vi "Stage Conditional Convert to TDMS.vi"(8 "error in (no error)":errorcluster, 11 "input cluster":T1={"Test_File"=path "", "Status"="Done", "RF_Center_Freq"=0.0, "RF_Gain"=0.0, "BB_Gain"=0.0, "Error 2"="", "file_max"=0, "file_index"=0}) -> (0 "error out":errorcluster, 2 "Converted Binary to TDMS location":path, 3 "output cluster":T1={"Test_File"=path "", "Status"="Done", "RF_Center_Freq"=0.0, "RF_Gain"=0.0, "BB_Gain"=0.0, "Error 2"="", "file_max"=0, "file_index"=0})   [LabVIEW 2017]
uses:
  TypeDef/ESC Internal Data Structure (types).ctl
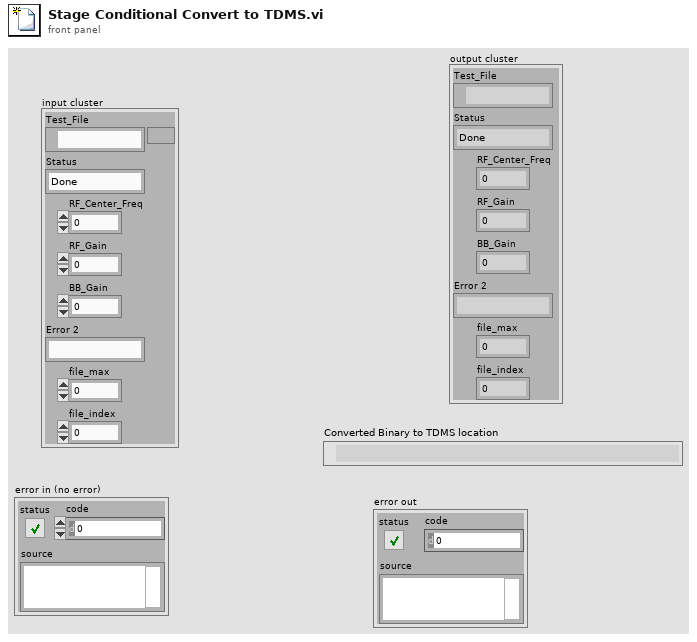
[diagram p1: front panel]
types:
  T1 = typedef "ESC Internal Data Structure (types).ctl" = cluster{"Test_File":path, "Status":string, "RF_Center_Freq":dbl, "RF_Gain":dbl, "BB_Gain":dbl, "Error 2":string, "file_max":u64, "file_index":u64}
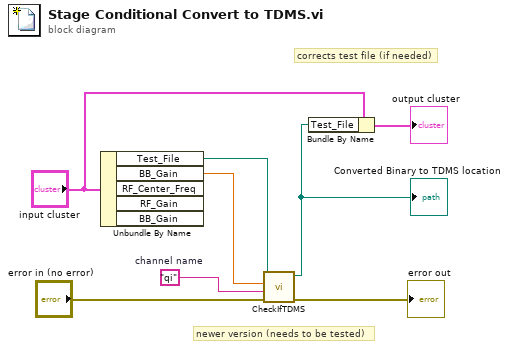
[diagram p0: block diagram]
diagram:
  w6 = "qi"  # channel name
  # "newer version (needs to be tested)"
  # "corrects test file (if needed)"
  n1 = Unbundle By Name("input cluster") -> ("Test_File"=w8:path, "BB_Gain"=w7:dbl)  [unwired: 3 out]
  n2 = call "CheckIfTDMS.vi"("error in (no error)"="error in (no error)", "channel name"=w6, "Scale Data"=w7, "original binary file Location"=w8) -> ("error out"=→"error out":errorcluster, "Converted Binary to TDMS location"=w2:path)  [unwired: 6 in]
  "Converted Binary to TDMS location" <- w2
  n3 = Bundle By Name(cluster="input cluster", "Test_File"=w2) -> (→"output cluster":T1)
